vi "Parse Bookmarks.vi"(8 "error in (no error)":errorcluster {"code" format="Error %.0f"}, 10 "VI Reference":refnum<vi>, 11 "VIDoc Parser In":refnum<class "VIDoc Parser.lvclass">) -> (0 "error out":errorcluster {"code" format="Error %.0f"}, 2 "Bookmarked?":bool, 3 "VIDoc Parser Out":refnum<class "VIDoc Parser.lvclass">)   [LabVIEW 2023, in "VIDoc Parsing.lvlib" / "VIDoc Parser.lvclass"]
uses:
  VIDoc Parser.lvclass
  VIDoc Parser.lvclass/VIDoc Parser.ctl
  <vilib>/Utility/miscctls.llb/LVMapReplaceAction.ctl
  Accessors/Get Parser Settings.vi
  Accessors/Get Bookmarks Map.vi
  GUI Documentation/GUI Documentation.lvclass
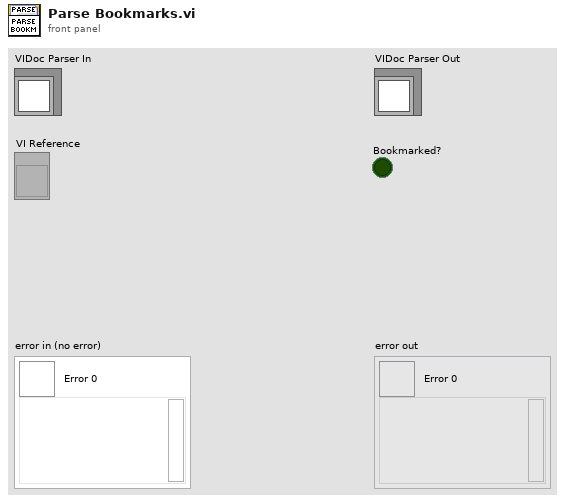
[diagram p1: front panel]
types:
  T1 = typedef "LVBookmarkInfoTypeDef.ctl" = cluster{"Bookmark Reference":u32, "Bookmark Tag":string, "Label Text":string}[]
  T2 = typedef "VIDoc Parsing.lvlib/Parser Settings.lvclass/Parser Settings Cluster.ctl" = cluster{"Draw Controls":T3, "Max Control Recursion Depth":i32, "Bookmarks Map":map{string, string[]}}
  T3 = typedef "VIDoc Parsing.lvlib/Parser Settings.lvclass/Draw Controls Cluster.ctl" = cluster{"Subpanels":bool, "Tabs":bool, "TypeDefs":bool, "Error Clusters":T4, "DVRs":T4, "Queues & Notifiers":T4}
  T4 = typedef "VIDoc Parsing.lvlib/Parser Settings.lvclass/Draw Option Enum.ctl" = enum16{"Ignore", "Draw", "Draw + Contents"}
  T5 = map{string, refnum<class "GUI Documentation.lvclass">[]}
  T6 = typedef "LVMapReplaceAction.ctl" = enum32{"Modify Entry only if found", "Add or Modify Entry", "Delete Entry"}
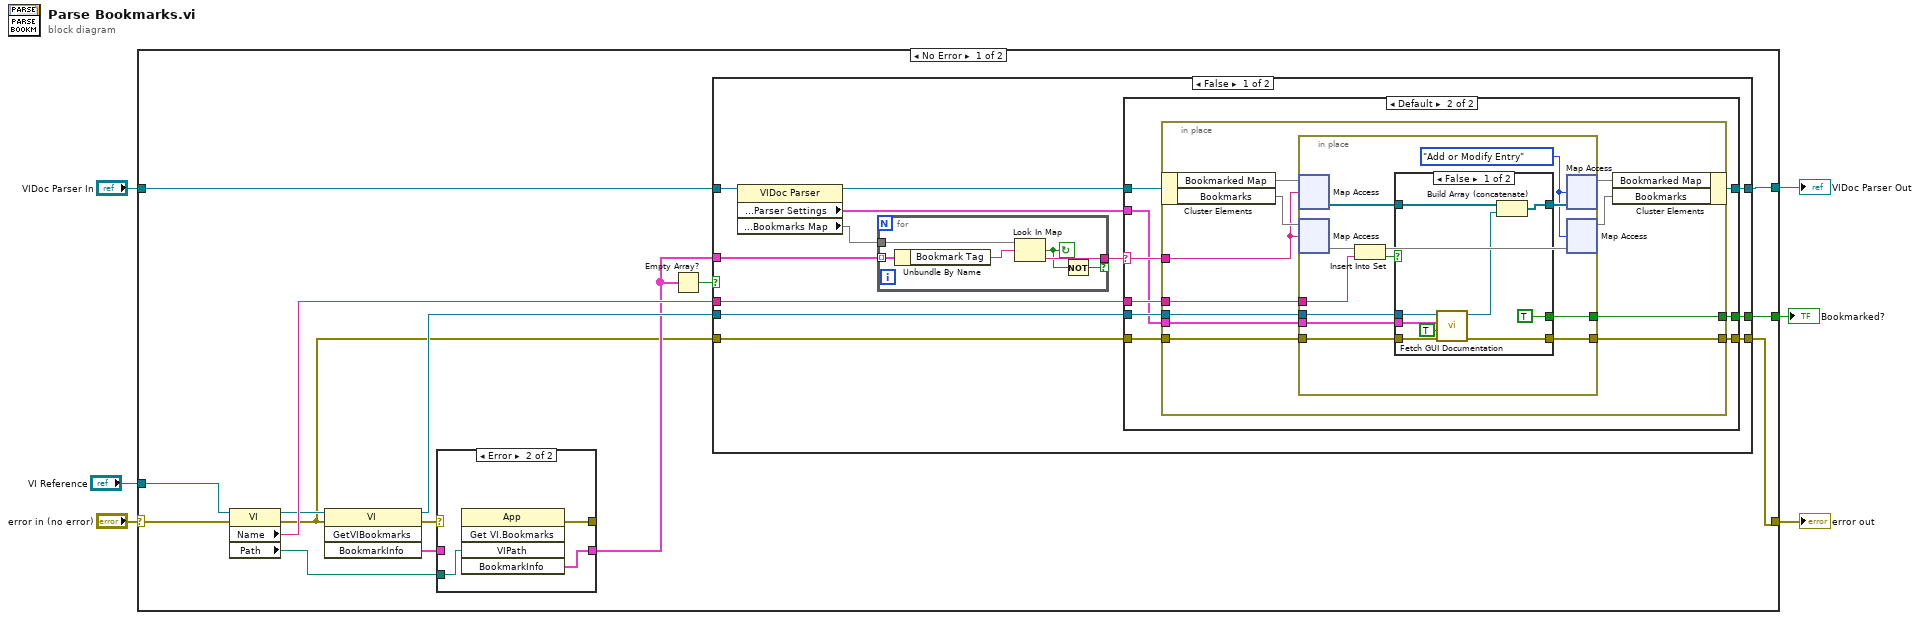
[diagram p0: block diagram]
diagram:
  n1 = case shown="No Error" "error in (no error)" {
    selector: "error in (no error)" -> [w19 w93]
    tunnel: [w17 w93] -> w5
    tunnel: [w20 w92] -> w3
    tunnel: "VIDoc Parser In" -> [w14 w92]
    tunnel: "VI Reference" -> [w18 _]
    tunnel: [w16 _] -> w1
    frame No Error {
      n2 = property class="VI"(reference=w18, error in=w19) -> (reference out=w11:refnum<vi>, error out=w8:errorcluster, "Name"=w15:string, "Path"=w7:path)
      n3 = invoke class="VI" method="GetVIBookmarks"(reference=w11, error in=w8) -> (reference out=w10:refnum<vi>, error out=w12:errorcluster, "BookmarkInfo"=w13:T1)  [unwired: 2 in, 1 out]
      n4 = case shown="Error" w12 {
        selector: w12 -> [w22 _]
        tunnel: w13 -> [w23 _]
        tunnel: [w23 w25] -> w9
        tunnel: [w22 w26] -> _
        tunnel: w7 -> [_ w24]
        frame No Error {
        }
        frame Error {
          n5 = invoke class="App" method="Get VI.Bookmarks"("VIPath"=w24) -> (error out=w26:errorcluster, "BookmarkInfo"=w25:T1)  [unwired: 4 in, 3 out]
        }
      }
      n6 = Empty Array?(array=w9) -> (empty?=w21:bool)
      n7 = case shown="False" w21 {
        tunnel: w9 -> [w37 _]
        tunnel: w14 -> [w28 w90]
        tunnel: [w38 w90] -> w20
        tunnel: w15 -> [w35 _]
        tunnel: w10 -> [w34 _]
        tunnel: w8 -> [w33 w91]
        tunnel: [w32 w91] -> w17
        tunnel: [w31 _] -> w16
        frame False {
          n8 = property class="VIDoc Parser"(reference=w28) -> (reference out=w27:refnum<class "VIDoc Parser.lvclass">, "Properties:Settings:Parser Settings"=w30:T2, "Properties:Settings:Bookmarks Map"=w29:map{string, string})  [unwired: 1 in, 1 out]
          n9 = for {
            tunnel: w37 -> [w44] mode=indexing
            tunnel: w29 -> [w43]
            tunnel: [w41] -> w36 if=w39
            stop <- w40 continue-if-true
            n10 = Unbundle By Name(w44) -> ("Bookmark Tag"=w42:string)
            n11 = Look In Map(map=w43, key=w42) -> (key not found?=w40:bool, value=w41:string)  [unwired: 1 in]
            n12 = Not(x=w40) -> (.not. x?=w39:bool)
          }
          n13 = case shown="Default" w36 {
            selector: w36 -> [_ w53]
            tunnel: w27 -> [w46 w55]
            tunnel: [w46 w54] -> w38
            tunnel: w30 -> [_ w50]
            tunnel: w35 -> [_ w52]
            tunnel: w34 -> [_ w51]
            tunnel: w33 -> [w45 w49]
            tunnel: [w45 w48] -> w32
            tunnel: [_ w47] -> w31
            frame "" {
            }
            frame Default {
              n14 = in-place "In Place Element Structure" {
                in-place-border: w53 -> [w64]
                in-place-border: w52 -> [w63]
                in-place-border: w51 -> [w62]
                in-place-border: w50 -> [w61]
                in-place-border: w49 -> [w60]
                in-place-border: [w59] -> w48
                in-place-border: [w56] -> w47
                n15 = in-place-cluster #1(w55) -> ("Bookmarked Map"=w66:T5, "Bookmarks"=w65:map{string, set{string}})
                n16 = in-place "In Place Element Structure" {
                  in-place-border: w63 -> [w75]
                  in-place-border: w62 -> [w72]
                  in-place-border: w61 -> [w71]
                  in-place-border: w60 -> [w70]
                  in-place-border: [w69] -> w59
                  in-place-border: [w67] -> w56
                  w68 = LVMapReplaceAction."Add or Modify Entry" ("action")
                  n17 = in-place-map #2(w66, w64) -> (w78:refnum<class "GUI Documentation.lvclass">[])  [unwired: 1 in, 1 out]
                  n18 = in-place-map #3(w65, w64) -> (w76:set{string})  [unwired: 1 in, 1 out]
                  n19 = Insert Into Set(10:w75, 11:w76) -> (2:w73:bool, 3:w74:set{string})
                  n20 = case shown="False" w73 {
                    tunnel: w78 -> [w86 w89]
                    tunnel: [w85 w89] -> w77
                    tunnel: w72 -> [w83 _]
                    tunnel: w71 -> [w82 _]
                    tunnel: w70 -> [w81 w88]
                    tunnel: [w80 w88] -> w69
                    tunnel: [TRUE _] -> w67
                    frame False {
                      n21 = call "Fetch GUI Documentation.vi"("error in (no error)"=w81, "Fetch Controls?"=TRUE, "Parser Settings"=w82, "VI Reference"=w83) -> ("error out"=w80:errorcluster, "GUI Documentation Out"=w84:refnum<class "GUI Documentation.lvclass">)  [unwired: 6 in]
                      n22 = Build Array (concatenate)(w86, w84) -> (w85:refnum<class "GUI Documentation.lvclass">[])
                    }
                    frame True {
                    }
                  }
                  n23 = in-place-map #2(w77, w68) -> (w58:T5)  [unwired: 2 out]
                  n24 = in-place-map #3(w74, w68) -> (w57:map{string, set{string}})  [unwired: 2 out]
                }
                n25 = in-place-cluster #1("Bookmarked Map"=w58, "Bookmarks"=w57) -> (w54:refnum<class "VIDoc Parser.lvclass">)
              }
            }
          }
        }
        frame True {
        }
      }
    }
    frame Error {
    }
  }
  "error out" <- w5
  "VIDoc Parser Out" <- w3
  "Bookmarked?" <- w1
